vi "PBPCIcard_start.vi"(0 "Base Address":u32 format="%.0x", 1 "Bytes/Word":u8=10, 2 "Memory":bool, 3 "error in (no error)":errorcluster) -> (7 "error out":errorcluster)   [LabVIEW 2013]
doc: "This vi sends a software trigger to the PulseBlaster.\n\nIn order to start the PulseBlaster, the following sequence must occur, even if the PulseBlaster is not reprogrammed, but merely retriggered:\n1) Reset the PulseBlaster\n2) Load number of bytes per word\n3) Select Memory device (external or internal)\n4) Clear address counter\n5) Send program finished\n6) Send the \"start\" trigger.\n\nThe inputs should rarely be changed, as they are hardware specific."
uses:
  pbcomm8.vi
  pbcomm16.vi
  pbcomm32.vi
panel:
  # "SOFTWARE TRIGGER"
  # "External"
  # "Internal"
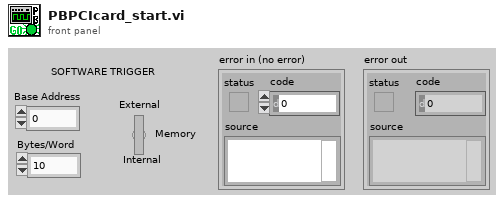
[diagram p1: front panel]
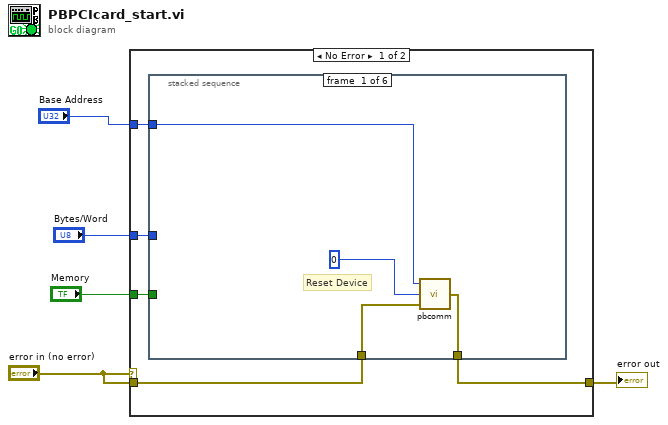
[diagram p0: block diagram]
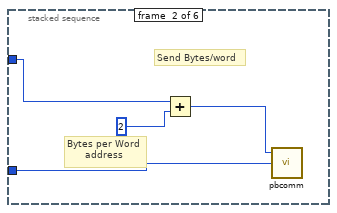
[diagram p2: hidden frame]
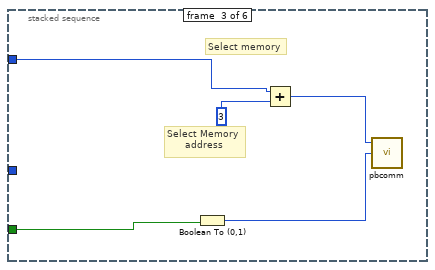
[diagram p3: hidden frame]
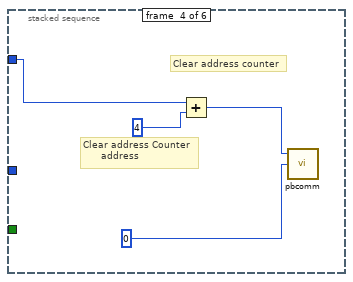
[diagram p4: hidden frame]
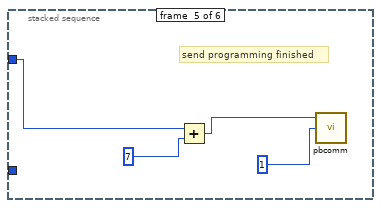
[diagram p5: hidden frame]
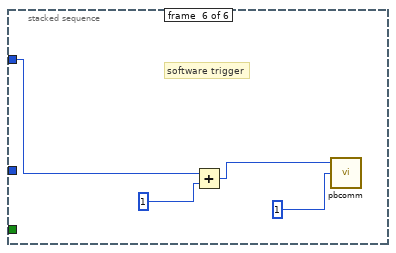
[diagram p6: hidden frame]
diagram:
  n1 = case shown="No Error" "error in (no error)" {
    tunnel: "Base Address" -> [w10 _]
    tunnel: "Bytes/Word" -> [w9 _]
    tunnel: "Memory" -> [w8 _]
    tunnel: [w6 w36] -> w1
    tunnel: "error in (no error)" -> [w7 w36]
    frame No Error {
      n2 = stacked-sequence {
        tunnel: w10 -> [w14 w16 w20 w24 w28 w32]
        tunnel: w9 -> [_ w15 _ _ _ _]
        tunnel: w8 -> [_ _ w19 _ _ _]
        tunnel: w7 -> [w12 _ _ _ _ _]
        tunnel: [w11 _ _ _ _ _] -> w6
        frame #0 {
          # "Reset Device"
          n3 = call-poly "pbcomm.vi"("error in"=w12, "write value"=u8 0, "address"=w14) -> ("error out"=w11:errorcluster)
        }
        frame #1 {
          # "Send Bytes/word"
          # "Bytes per Word\n      address"
          n4 = Add(x=w16, y=u8 2) -> (x+y=w17:u32)
          n5 = call-poly "pbcomm.vi"("write value"=w15, "address"=w17) -> ()  [unwired: 1 in, 1 out]
        }
        frame #2 {
          # "Select memory"
          # "Select Memory\n      address"
          n6 = Boolean To (0,1)(Boolean=w19) -> (0, 1=w21:i16)
          n7 = Add(x=w20, y=u8 3) -> (x+y=w22:u32)
          n8 = call-poly "pbcomm.vi"("write value"=w21, "address"=w22) -> ()  [unwired: 1 in, 1 out]
        }
        frame #3 {
          # "Clear address counter"
          # "Clear address Counter\n      address"
          n9 = Add(x=w24, y=u8 4) -> (x+y=w26:u32)
          n10 = call-poly "pbcomm.vi"("write value"=u8 0, "address"=w26) -> ()  [unwired: 1 in, 1 out]
        }
        frame #4 {
          # "send programming finished"
          n11 = Add(x=w28, y=7) -> (x+y=w30:u32)
          n12 = call-poly "pbcomm.vi"("write value"=1, "address"=w30) -> ()  [unwired: 1 in, 1 out]
        }
        frame #5 {
          # "software trigger"
          n13 = Add(x=w32, y=1) -> (x+y=w34:u32)
          n14 = call-poly "pbcomm.vi"("write value"=1, "address"=w34) -> ()  [unwired: 1 in, 1 out]
        }
      }
    }
    frame Error {
    }
  }
  "error out" <- w1
